vi "Drive Forward Drive.vi"(8 "error in (no error)":errorcluster, 10 "Joystick State":T1, 11 "Comp Driver in":refnum<class "Comp Driver.lvclass">) -> (0 "error out":errorcluster, 3 "Comp Driver out":refnum<class "Comp Driver.lvclass">)   [LabVIEW 2014, in "Comp Driver.lvlib" / "Comp Driver.lvclass"]
uses:
  Comp Driver.lvclass
  Robot/Joystick/Joystick Class/Joystick State.ctl
  Robot/Joystick/Joystick Class/Button State.ctl
  Robot/Joystick/Joystick Class/Axis State.ctl
  Robot/Driver/Driver Class/Driver.lvclass
  Robot/Joystick/Joystick Class/Joystick.lvclass
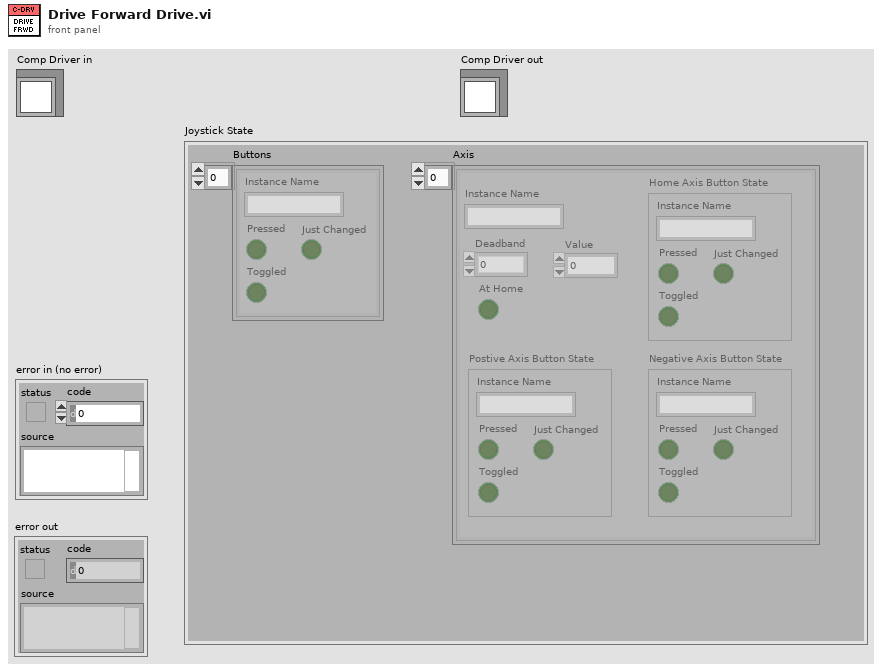
[diagram p1: front panel]
types:
  T1 = typedef "Joystick.lvlib/Joystick.lvclass/Joystick State.ctl" = cluster{"Buttons":T2[], "Axis":T3[]}
  T2 = typedef "Joystick.lvlib/Joystick.lvclass/Button State.ctl" = cluster{"Pressed":bool, "Instance Name":string, "Toggled":bool, "Just Changed":bool}
  T3 = typedef "Joystick.lvlib/Joystick.lvclass/Axis State.ctl" = cluster{"Instance Name":string, "Deadband":dbl, "Value":dbl, "At Home":bool, "Postive Axis Button State":T2, "Negative Axis Button State":T2, "Home Axis Button State":T2}
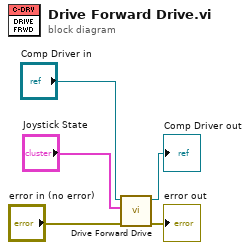
[diagram p0: block diagram]
diagram:
  n1 = call-parent "Drive Forward Drive.vi"("error in (no error)"="error in (no error)", "Joystick State"="Joystick State", "Driver in"="Comp Driver in") -> ("error out"=→"error out":errorcluster, "Driver out"=→"Comp Driver out":refnum<class "Comp Driver.lvclass">)  [unwired: 7 in]
